vi "TW Update Project Internal Paths.vi"(7 "Rename Project":bool=TRUE, 8 "error in (no error)":errorcluster, 9 "Replace Subname":string="Template", 10 "New Subname":string, 11 "Project Path":path) -> (0 "error out":errorcluster)   [LabVIEW 2021, in "LV Scripting Utilities.lvlib"]
uses:
  LV Scripting Utilities.lvlib
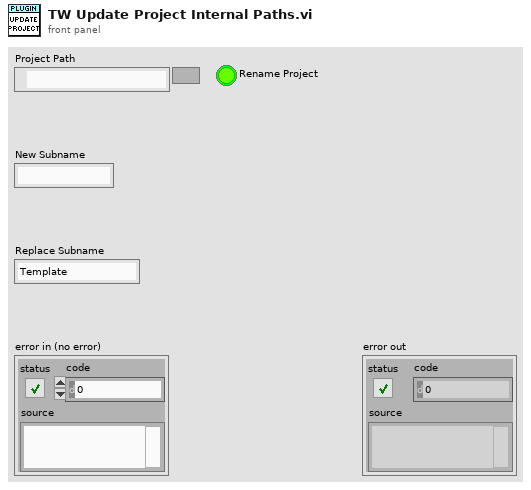
[diagram p1: front panel]
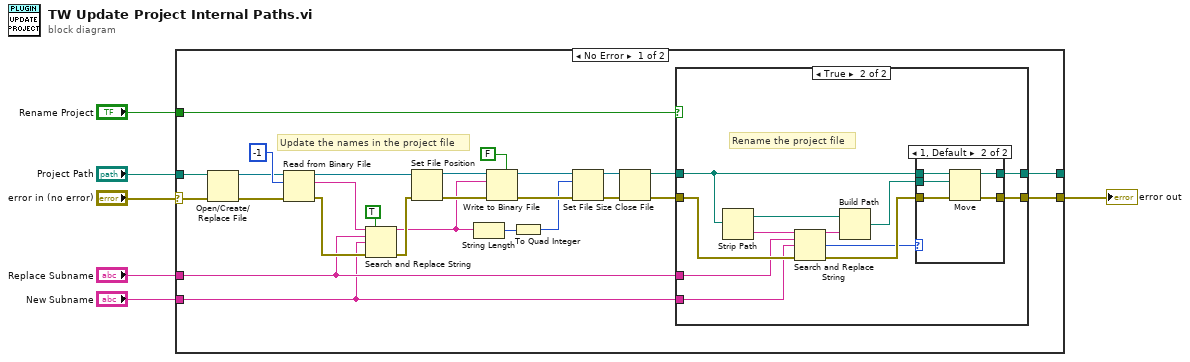
[diagram p0: block diagram]
diagram:
  n1 = case shown="No Error" "error in (no error)" {
    selector: "error in (no error)" -> [w20 w55]
    tunnel: [w25 w55] -> w1
    tunnel: [w24 _] -> _
    tunnel: "Project Path" -> [w19 _]
    tunnel: "New Subname" -> [w14 _]
    tunnel: "Replace Subname" -> [w15 _]
    tunnel: "Rename Project" -> [w16 _]
    frame No Error {
      # "Update the names in the project file"
      n2 = Open/Create/Replace File(file path (use dialog)=w19, error in=w20) -> (refnum out=w21:refnum<file>, error out=w23:errorcluster)  [unwired: 4 in, 1 out]
      n3 = Read from Binary File(8:w23, 10:-1 ("count (1)"), 11:w21) -> (0:w18:errorcluster, 2:w33:string, 3:w30:refnum<file>)  [unwired: 3 in, 1 out]
      n4 = Search and Replace String(replace all?=TRUE ("replace all? (F)"), input string=w33, search string=w15, replace string=w14, error in=w18) -> (result string=w9:string, error out=w17:errorcluster)  [unwired: 3 in, 2 out]
      n5 = Set File Position(refnum=w30, error in=w17) -> (refnum out=w29:refnum<file>, error out=w28:errorcluster)  [unwired: 2 in]
      n6 = String Length(string=w9) -> (length=w8:i32)
      n7 = Write to Binary File(file (use dialog)=w29, data=w9, error in=w28, 5:FALSE ("prepend array or string size? (T)")) -> (refnum out=w13:refnum<file>, error out=w12:errorcluster)  [unwired: 2 in, 1 out]
      n8 = To Quad Integer(1:w8) -> (0:w7:i64)
      n9 = Set File Size(4:w12, 6:w7, 7:w13) -> (0:w11:errorcluster, 3:w10:refnum<file>)
      n10 = Close File(refnum=w10, error in=w11) -> (path=w26:path, error out=w27:errorcluster)
      n11 = case shown="True" w16 {
        tunnel: w27 -> [w34 w42]
        tunnel: w26 -> [w35 w46]
        tunnel: [w34 w44] -> w25
        tunnel: [w35 w43] -> w24
        tunnel: w14 -> [_ w38]
        tunnel: w15 -> [_ w37]
        frame False {
        }
        frame True {
          # "Rename the project file"
          n12 = Strip Path(path=w46) -> (stripped path=w47:path, name=w40:string)
          n13 = Search and Replace String(input string=w40, search string=w37, replace string=w38, error in=w42) -> (result string=w39:string, number of replacements=w36:i32, error out=w41:errorcluster)  [unwired: 4 in, 1 out]
          n14 = Build Path(base path=w47, name or relative path=w39) -> (appended path=w45:path)
          n15 = case shown="1, Default" w36 {
            tunnel: w46 -> [w49 w54]
            tunnel: w45 -> [_ w53]
            tunnel: [w48 w52] -> w44
            tunnel: [w49 w51] -> w43
            tunnel: w41 -> [w48 w50]
            frame 0 {
            }
            frame 1, Default {
              n16 = Move(source path=w54, error in=w50, 10:w53) -> (error out=w52:errorcluster, 3:w51:path)  [unwired: 2 in, 1 out]
            }
          }
        }
      }
    }
    frame Error {
    }
  }
  "error out" <- w1
